vi "FTW-Actor-ValidateAddress.vi"(5 "Address":string, 7 "Allow wildcard replacement?":bool, 11 "error in":errorcluster) -> (6 "Sanitized Address":string, 8 "Message Transport Scheme":T1, 15 "error out":errorcluster)   [LabVIEW 2012, in "FTW-Actor.lvlib"]
uses:
  FTW-Actor.lvlib
  Endpoint/FTW-Endpoint-MessageTransportScheme.ctl
  Endpoint/FTW-Endpoint.lvclass
panel:
  # "Inputs"
  # "Outputs"
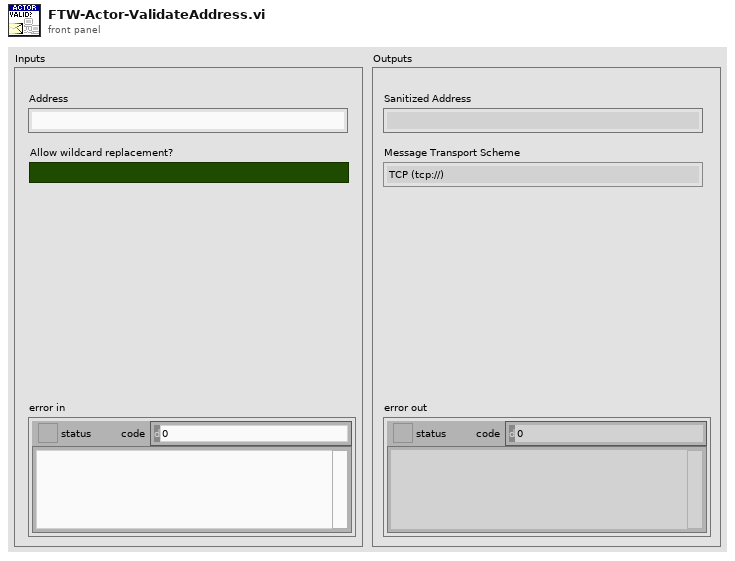
[diagram p1: front panel]
types:
  T1 = typedef "FTW-Actor.lvlib/FTW-Endpoint.lvclass/FTW-Endpoint-MessageTransportScheme.ctl" = enum16{"TCP (tcp://)", "Inter-Process (ipc://)", "In-Process (inproc://)"}
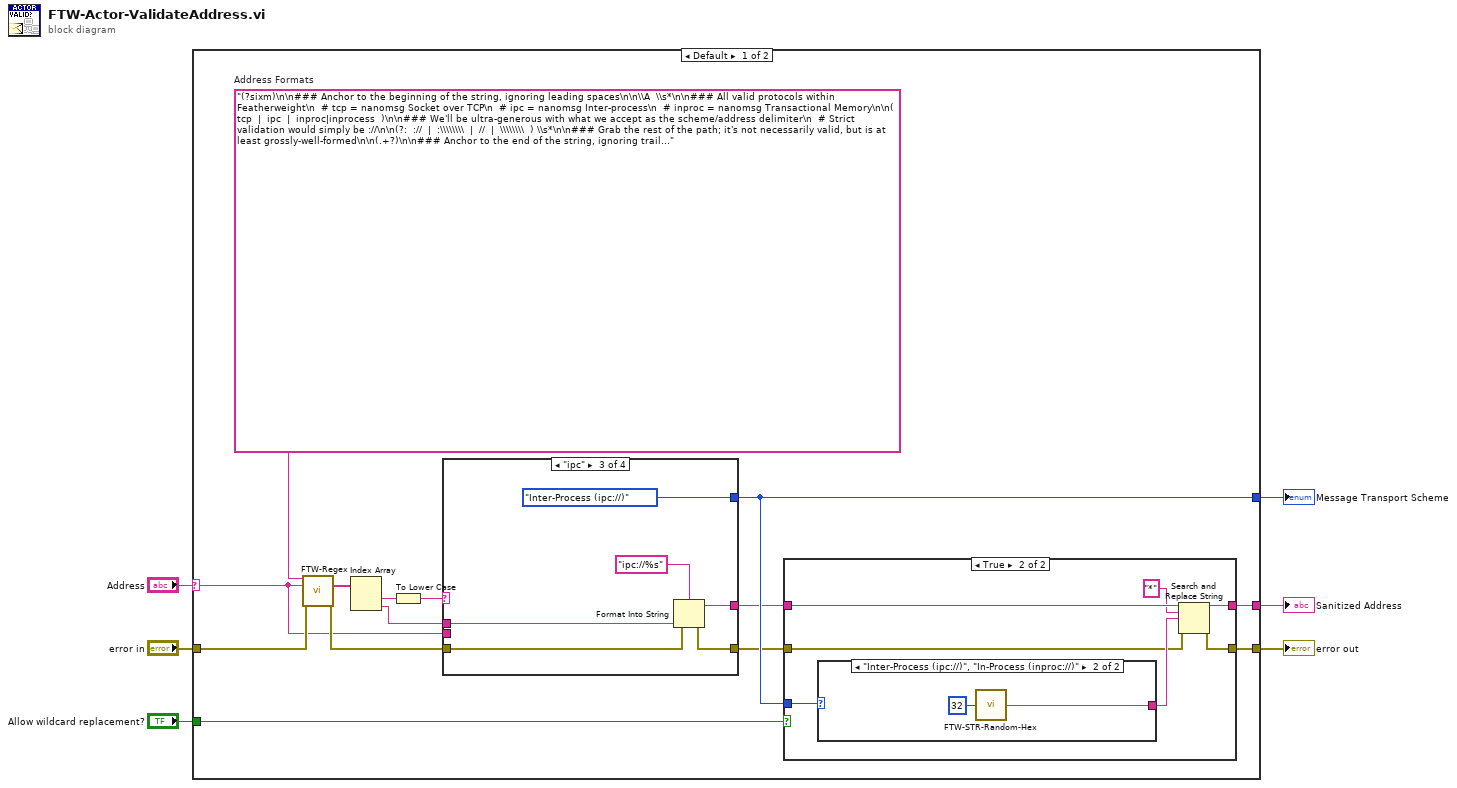
[diagram p0: block diagram]
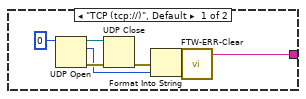
[diagram p3: hidden frame]
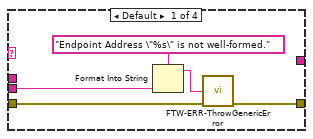
[diagram p4: hidden frame]
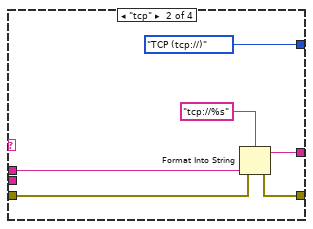
[diagram p5: hidden frame]
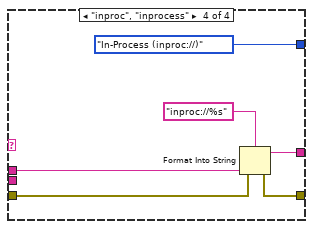
[diagram p6: hidden frame]
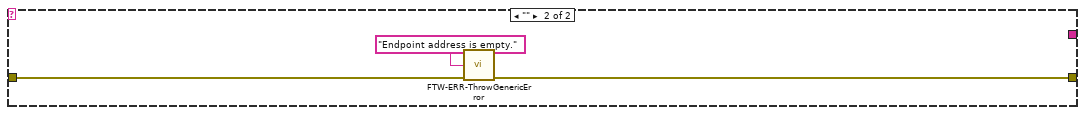
[diagram p7: hidden frame]
diagram:
  n1 = case shown="Default" "Address" {
    selector: "Address" -> [w13 _]
    tunnel: "error in" -> [w18 w64]
    tunnel: [w12 _] -> w5
    tunnel: [w8 _] -> w4
    tunnel: [w9 w63] -> w3
    tunnel: "Allow wildcard replacement?" -> [w7 _]
    frame Default {
      w20 = "(?sixm)\n\n### Anchor to the beginning of the string, ignoring leading spaces\n\n\\A  \\s*\n\n### All valid protocols within Featherweight\n  # tcp = nanomsg Socket over TCP\n  # ipc = nanomsg Inter-process\n  # inproc = nanomsg Transactional Memory\n\n(  tcp  |  ipc  |  inproc|inprocess  )\n\n### We'll be ultra-generous with what we accept as the scheme/address delimiter\n  # Strict validation would simply be ://\n\n(?:  ://  |  :\\\\\\\\  |  //  |  \\\\\\\\  ) \\s*\n\n### Grab the rest of the path; it's not necessarily valid, but is at least grossly-well-formed\n\n(.+?)\n\n### Anchor to the end of the string, ignoring trailing spaces\n\\s*\\z"  # Address Formats
      n2 = call "FTW-Regex.vi"("Regular Expression"=w20, "Input String"=w13, "error in"=w18) -> ("Submatches"=w19:string[], "error out"=w15:errorcluster)  [unwired: 8 in, 3 out]
      n3 = Index Array(array=w19) -> (element #1=w17:string, element #2=w14:string)  [unwired: 2 in]
      n4 = To Lower Case(string=w17) -> (all lower case string=w16:string)
      n5 = case shown="\"ipc\"" w16 {
        tunnel: [_ FTW-Endpoint-MessageTransportScheme."TCP (tcp://)" ("Message Transport Scheme") FTW-Endpoint-MessageTransportScheme."Inter-Process (ipc://)" ("Message Transport Scheme") FTW-Endpoint-MessageTransportScheme."In-Process (inproc://)" ("Message Transport Scheme")] -> w12
        tunnel: w15 -> [w41 w44 w50 w56]
        tunnel: w13 -> [w40 _ _ _]
        tunnel: [w39 w46 w52 w58] -> w10
        tunnel: w14 -> [_ w45 w51 w57]
        tunnel: [_ w47 w53 w59] -> w11
        frame Default {
          n6 = Format Into String(format string="Endpoint Address \"%s\" is not well-formed." ("Error Message"), w40) -> (resulting string=w43:string)  [unwired: 2 in, 1 out]
          n7 = call "FTW-ERR-ThrowGenericError.vi"("Error Message"=w43, "error in"=w41) -> ("error out"=w39:errorcluster)  [unwired: 13 in]
        }
        frame "tcp" {
          n8 = Format Into String(format string="tcp://%s", error in=w44, w45) -> (resulting string=w47:string, error out=w46:errorcluster)  [unwired: 1 in]
        }
        frame "ipc" {
          n9 = Format Into String(format string="ipc://%s", error in=w50, w51) -> (resulting string=w53:string, error out=w52:errorcluster)  [unwired: 1 in]
        }
        frame "inproc", "inprocess" {
          n10 = Format Into String(format string="inproc://%s", error in=w56, w57) -> (resulting string=w59:string, error out=w58:errorcluster)  [unwired: 1 in]
        }
      }
      n11 = case shown="True" w7 {
        tunnel: w12 -> [_ w29]
        tunnel: w11 -> [w22 w27]
        tunnel: w10 -> [w21 w26]
        tunnel: [w21 w25] -> w9
        tunnel: [w22 w24] -> w8
        frame False {
        }
        frame True {
          n12 = case shown="\"Inter-Process (ipc://)\", \"In-Process (inproc://)\"" w29 {
            tunnel: [w30 w37] -> w28
            frame "TCP (tcp://)", Default {
              n13 = UDP Open(11:u16 0 ("port")) -> (port=w35:refnum<k16>, 0:w34:errorcluster, 2:w32:u16)  [unwired: 4 in]
              n14 = UDP Close(connection ID=w35, 8:w34) -> (error out=w33:errorcluster)  [unwired: 1 out]
              n15 = Format Into String(error in=w33, w32) -> (resulting string=w30:string, error out=w31:errorcluster)  [unwired: 2 in]
              n16 = call "FTW-ERR-Clear.vi"("error to snuff"=w31) -> ()  [unwired: 1 out]
            }
            frame "Inter-Process (ipc://)", "In-Process (inproc://)" {
              n17 = call "FTW-STR-Random-Hex.vi"("String Length"=32) -> ("Random Hex String"=w37:string)  [unwired: 3 in]
            }
          }
          n18 = Search and Replace String(input string=w27, search string="*", replace string=w28, error in=w26) -> (result string=w24:string, error out=w25:errorcluster)  [unwired: 4 in, 2 out]
        }
      }
    }
    frame "" {
      n19 = call "FTW-ERR-ThrowGenericError.vi"("Error Message"="Endpoint address is empty.", "error in"=w64) -> ("error out"=w63:errorcluster)  [unwired: 13 in]
    }
  }
  "error out" <- w3
  "Message Transport Scheme" <- w5
  "Sanitized Address" <- w4
